vi "rs3 Advanced set RAU control3.vi"(8 "error in (no error)":errorcluster, 10 "ST RAU vector":T1, 11 "device in":u64) -> (0 "error out":errorcluster, 1 "error":u64, 3 "Dev out":u64)   [LabVIEW 2018, in "libRealSense3.lvlib"]
doc: "This sets some register that affect the depth calculations"
uses:
  libRealSense3.lvlib
  realsense2.dll
panel:
  # "RS2 Adv. Set RAU"
  # "(C) 2017 Intel Corp.,  AGJ"
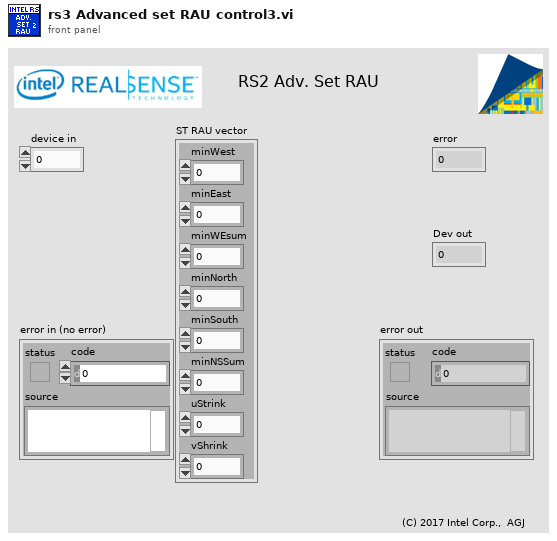
[diagram p1: front panel]
types:
  T1 = cluster{"minWest":u32, "minEast":u32, "minWEsum":u32, "minNorth":u32, "minSouth":u32, "minNSSum":u32, "uStrink":u32, "vShrink":u32}
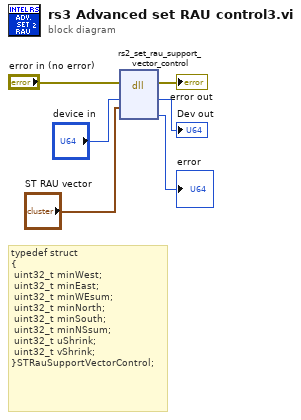
[diagram p0: block diagram]
diagram:
  # "typedef struct\n{\n\tuint32_t minWest;\n\tuint32_t minEast;\n\tuint32_t minWEsum;\n\tuint32_t minNorth;\n\tuint32_t minSouth;\n\tuint32_t minNSsum;\n\tuint32_t uShrink;\n\tuint32_t vShrink;\n}STRauSupportVectorControl;"
  n1 = dll-call lib="C:/Users/aaron.jencks/Documents/GitHub/emerson_seed_object_detection/LabVIEW/Projects/Paul's Video Viewer/Classes/Realsense Cam/realsense_wrapper_api/realsense2.dll" fn="rs2_set_rau_support_vector_control"(error in="error in (no error)", "device"="device in", "ST RAU vector"="ST RAU vector") -> (error out=→"error out":errorcluster, "device"=→"Dev out":u64, "error"=→"error":u64)  [unwired: 5 in, 1 out]
